vi "Perform crosstalk measurement.vi"(8 "error in (no error)":errorcluster, 10 "I2S waveforms":waveform(dbl)[](array[waveform]), 11 "measurement configuration":T2={"Weighting filter"="Linear", "Full scale range"=2.825, "Channel name"="", "Analog source resource name"="", "Frequency"=0.0, "Amplitude"=0.0, "Protocol capture resource name"="", "Data line"=0, "Interferer channel"=0, "Victim channel"=0, "Sample rate"=44100.0, "Measurement duration"=0.1, "Frame sync edge for channel 0"=1, "Channel count per frame"=2, "Channel length"=32, "Bit depth"=24, "Channel 0 offset"=1, "Endianness"=0, "Data justification"=0, "Frame length"=64, "Frame sync pulse width"=32, "Bit clock edge sync"=1}) -> (0 "error out":errorcluster, 3 "measurement results":T1)   [LabVIEW 2021, in "crosstalk_Audio ADC.lvlib"]
uses:
  crosstalk_Audio ADC.lvlib
  Measurement Configuration.ctl
  Measurement Results.ctl
  <vilib>/addons/_NISVFA/_Shared subVIs/Common/SVL Set dB Reference (N Ch - 1 Ref).vi
  <vilib>/addons/_NISVFA/_Spectrum Processing/SVFA Unit Conversion (Complex) (1 Ch).vi
  <vilib>/addons/_NISVFA/_Shared subVIs/Common/SVL Set dB Reference (1 Ch).vi
  <vilib>/addons/_NISVFA/_Shared subVIs/Common/svc_Log View for Spectrum (1Ch).vi
  <vilib>/addons/_NISVFA/_Spectrum Processing/SVFA Unit Conversion (1 Ch).vi
  <vilib>/addons/_NISVFA/_Shared subVIs/Common/svc_Complex Datatype Defaults.vi
  <vilib>/addons/_NISVFA/_Shared subVIs/Common/SVL Set dB Reference (variant).vi
  <vilib>/addons/_NISVFA/_Shared subVIs/Common/svc_Unwrap Phase.vi
  <vilib>/addons/_NISVFA/_Shared subVIs/Common/svc_Convert Spectrum Array to dB.vi
  <vilib>/addons/_NISVFA/_Shared subVIs/Common/svc_Spectrum Units.vi
  <vilib>/addons/_NISVFA/_Spectrum Processing/subVIs/svfa_Conversion Utility (spectrum info).vi
  <vilib>/addons/_NISVFA/_Shared subVIs/Common/svc_Format Value (DBL).vi
  <vilib>/addons/_NISVFA/_Shared subVIs/Common/svc_Get Weighting Enum and Labels.vi
  <vilib>/addons/_NISVFA/_Shared subVIs/Common/svc_Engineering Units to Unit Label.vi
  <vilib>/addons/_NISVFA/_Shared subVIs/Common/svc_Surround NonAlpha String with Parentheses.vi
  <vilib>/dlg_ctls.llb/Space Constant.vi
  <vilib>/addons/_NISVFA/_Spectrum Processing/subVIs/svfa_Peak to RMS to Peak2Peak.vi
  <vilib>/addons/_NISVFA/_Spectrum Processing/subVIs/svfa_Mag to Mag2.vi
  <vilib>/addons/_NISVFA/_Spectrum Processing/subVIs/svfa_Linear to dB.vi
  <vilib>/addons/_NISVFA/_Spectrum Processing/subVIs/svfa_dBrefA to dBrefB.vi
  <vilib>/addons/_NISVFA/_Spectrum Processing/subVIs/svfa_Spectrum to Spectral Density.vi
  <vilib>/addons/_NISVFA/_Shared subVIs/Common/svc_Unit Label Lexical Class.vi
  <vilib>/addons/_NISVFA/_Shared subVIs/Common/svc_Window Parameters.vi
  <vilib>/addons/_NISVFA/_Shared subVIs/Common/svc_Caller VI Returned in Error Source.vi
  <vilib>/addons/Sound and Vibration/svt_Single Tone Measurements/SVT Crosstalk (Time).vi
  <vilib>/Analysis/4window.llb/window parameters.vi
  <vilib>/Analysis/4window.llb/Window Properties.vi
  <vilib>/Analysis/4window.llb/Window Properties by Name.vi
  <vilib>/addons/Sound and Vibration/svt_Single Tone Measurements/SoundVib_SingleTone.lvlib
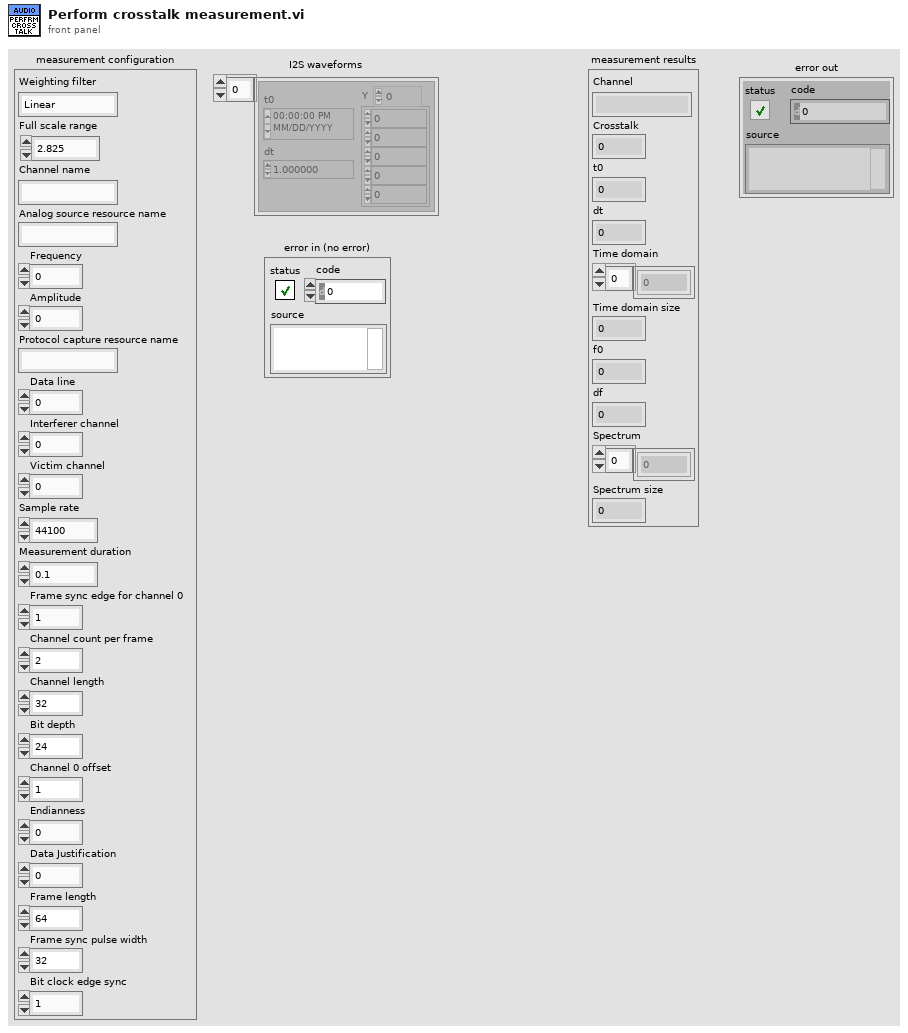
[diagram p1: front panel]
types:
  T1 = typedef "Crosstalk_Audio ADC.lvlib/Measurement Results.ctl" = cluster{"Channel":string, "Crosstalk":dbl, "t0":dbl, "dt":dbl, "Time domain":dbl[], "Time domain size":u32, "f0":dbl, "df":dbl, "Spectrum":dbl[], "Spectrum size":u32}
  T2 = typedef "Crosstalk_Audio ADC.lvlib/Measurement Configuration.ctl" = cluster{"Weighting filter":string, "Full scale range":dbl, "Channel name":string, "Analog source resource name":string, "Frequency":dbl, "Amplitude":dbl, "Protocol capture resource name":string, "Data line":u32, "Interferer channel":u32, "Victim channel":u32, "Sample rate":dbl, "Measurement duration":dbl, "Frame sync edge for channel 0":u32, "Channel count per frame":u32, "Channel length":u32, "Bit depth":u32, "Channel 0 offset":u32, "Endianness":u32, "Data justification":u32, "Frame length":u32, "Frame sync pulse width":u32, "Bit clock edge sync":u32}
  T3 = cluster{"linear/dB":enum16{"no change", "linear", "dB"}, "dB reference (0: no change)":dbl, "power/magnitude":enum16{"no change", "power", "magnitude"}, "view":enum16{"no change", "rms", "peak", "peak-peak"}}
  T4 = typedef "svc_Spectrum Info.ctl" = cluster{"channel name":string, "description":string, "x-axis units":T5, "spectral info":cluster{"spectrum type":T6, "linear/dB":enum16{"linear", "dB"}, "window":u16, "window size":i32, "FFT size":i32}, "engineering units":T7, "custom label":string, "dB reference [EU]":dbl, "peak units":enum16{"rms", "peak", "peak-peak"}, "weighting filter":T8, "spectral density?":bool, "unit label":string, "spectrum skewed?":bool, "complimentary spectrum units":T9}
  T5 = typedef "svc_X-Axis Units.ctl" = u16
  T6 = typedef "svc_Spectrum Type.ctl" = enum16{"FFT Spectrum [complex]", "Amplitude [Magnitude]", "Power [Magnitude^2]", "Cross Spectrum [complex]", "Frequency Response [Complex]"}
  T7 = typedef "svc_Engineering Units Text Ring.ctl" = u16
  T8 = typedef "svc_Weighting Filter Text Ring.ctl" = u16
  T9 = typedef "svc_Complimentary Spectrum Units.ctl" = enum16{"none", "radians", "degrees", "cycles", "imaginary"}
  T10 = cluster{"complex spectrum response":cluster{"f0":dbl, "df":dbl, "complex spectrum":cdb[]}, "spectrum info":T4}
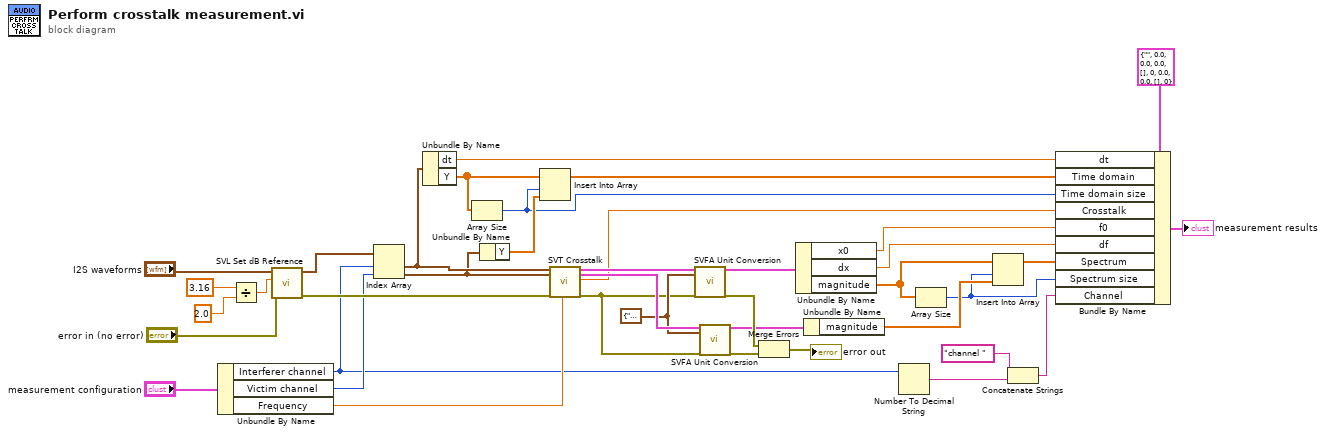
[diagram p0: block diagram]
diagram:
  w27 = T3 {"linear/dB"=enum."dB", "dB reference (0: no change)"=0.0, "power/magnitude"=enum."magnitude", "view"=enum."peak"} ("desired scaling")
  n1 = Unbundle By Name("measurement configuration") -> ("Interferer channel"=w8:u32, "Victim channel"=w33:u32, "Frequency"=w29:dbl)
  n2 = Divide(x=3.16, y=2.0) -> (x/y=w30:dbl)
  n3 = call-poly <vilib>:"SVL Set dB Reference.vi"("error in (no error)"="error in (no error)", "dB reference [EU]"=w30, "scaled signals in [EU]"="I2S waveforms") -> ("error out"=w35:errorcluster, "scaled signals out [EU]"=w36:waveform(dbl)[])  [unwired: 7 in]
  n4 = Index Array(array=w36, index #1=w8, index #2=w33) -> (element #1=w15:waveform(dbl), element #2=w12:waveform(dbl))
  n5 = Unbundle By Name ("Get Waveform Components")(w15) -> ("dt"=w14:dbl, "Y"=w13:dbl[])
  n6 = Array Size(array=w13) -> (size(s)=w9:i32)
  n7 = Unbundle By Name ("Get Waveform Components")(w12) -> ("Y"=w11:dbl[])
  n8 = Insert Into Array(array=w13, index=w9, new element=w11) -> (w10:dbl[])
  n9 = call-poly <vilib>:"SVT Crosstalk.vi"("stimulus signal X [EUx]"=w15, "idle-channel response signal Y [EUy]"=w12, "error in (no error)"=w35, "expected fundamental frequency [Hz]"=w29) -> ("complex spectrum\nstimulus X"=w39:T10, "complex spectrum\nidle-channel response Y"=w28:T10, "crosstalk"=w16:dbl, "error out"=w26:errorcluster)  [unwired: 8 in, 4 out]
  n10 = call-poly <vilib>:"SVFA Unit Conversion.vi"("complex spectrum"=w39, "desired scaling"=w27, "error in (no error)"=w26) -> ("converted spectrum"=w24:cluster{"x0":dbl, "dx":dbl, "magnitude":dbl[]}, "error out"=w37:errorcluster)  [unwired: 11 in, 4 out]
  n11 = call-poly <vilib>:"SVFA Unit Conversion.vi"("complex spectrum"=w28, "desired scaling"=w27, "error in (no error)"=w26) -> ("converted spectrum"=w23:cluster{"x0":dbl, "dx":dbl, "magnitude":dbl[]}, "error out"=w38:errorcluster)  [unwired: 11 in, 4 out]
  n12 = Merge Errors(w37, w38) -> (→"error out":errorcluster)
  n13 = Unbundle By Name(w24) -> ("x0"=w19:dbl, "dx"=w18:dbl, "magnitude"=w22:dbl[])
  n14 = Unbundle By Name(w23) -> ("magnitude"=w21:dbl[])
  n15 = Number To Decimal String(number=w8) -> (decimal integer string=w7:string)  [unwired: 1 in]
  n16 = Array Size(array=w22) -> (size(s)=w17:i32)
  n17 = Insert Into Array(array=w22, index=w17, new element=w21) -> (w20:dbl[])
  n18 = Concatenate Strings("channel " ("string"), w7) -> (w5:string)
  n19 = Bundle By Name(cluster=T1 {"Channel"="", "Crosstalk"=0.0, "t0"=0.0, "dt"=0.0, "Time domain"=[], "Time domain size"=0, "f0"=0.0, "df"=0.0, "Spectrum"=[], "Spectrum size"=0} ("measurement results"), "dt"=w14, "Time domain"=w10, "Time domain size"=w9, "Crosstalk"=w16, "f0"=w19, "df"=w18, "Spectrum"=w20, "Spectrum size"=w17, "Channel"=w5) -> (→"measurement results":T1)
